vi "JSON to Waveform.vi"(11 "message":string) -> (3 "Waveform":waveform(dbl))   [LabVIEW 2016]
uses:
  <vilib>/addons/_JKI.lib/Serialization/JSON/Deserializer/JSON Deserializer/JSON Deserializer.lvclass
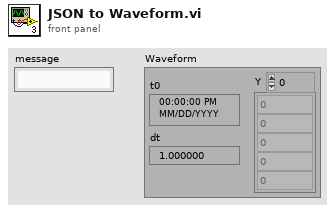
[diagram p1: front panel]
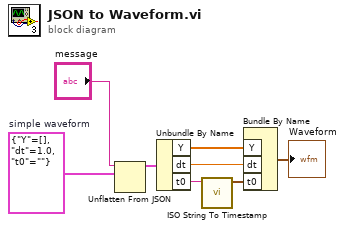
[diagram p0: block diagram]
diagram:
  w8 = cluster{"Y":dbl[], "dt":dbl, "t0":string} {"Y"=[], "dt"=1.0, "t0"=""}  # simple waveform
  n1 = Unflatten From JSON(JSON string="message", type and defaults=w8) -> (value=w4:cluster{"Y":dbl[], "dt":dbl, "t0":string})  [unwired: 5 in, 1 out]
  n2 = Unbundle By Name(w4) -> ("Y"=w5:dbl[], "dt"=w6:dbl, "t0"=w2:string)
  n3 = call <vilib>:"ISO String To Timestamp.vi"("ISO Timestamp String"=w2) -> ("Time Stamp"=w1:timestamp)  [unwired: 9 in, 1 out]
  n4 = Bundle By Name("Y"=w5, "dt"=w6, "t0"=w1) -> (→"Waveform":waveform(dbl))  [unwired: 1 in]
